vi "Cluster Terminal Get Elements Info.vi"(7 "skip first typedef?":bool, 8 "error in (no error)":errorcluster, 10 "ClusterConstant refnum":refnum<vi>, 11 "Terminal in":refnum<vi>) -> (0 "error out":errorcluster, 1 "is typedef?":bool, 2 "Cluster elements datatypes":string[](array[string]), 3 "Cluster elements names":string[](array[string]), 4 "typedef name":string)   [LabVIEW 2014]
doc: "Returns names and datatypes of elements inside cluster. If elemnet has no label, it's returned default name \"item0\" or \"item1\" or ... \"itemN\" which will be also used in generated code.\nIf wired Terminal then is used to get names and datatypes of ClusterConstant elements, otherwise is used ClusterConstant refnum."
uses:
  TranscriptorBasicObject.lvclass
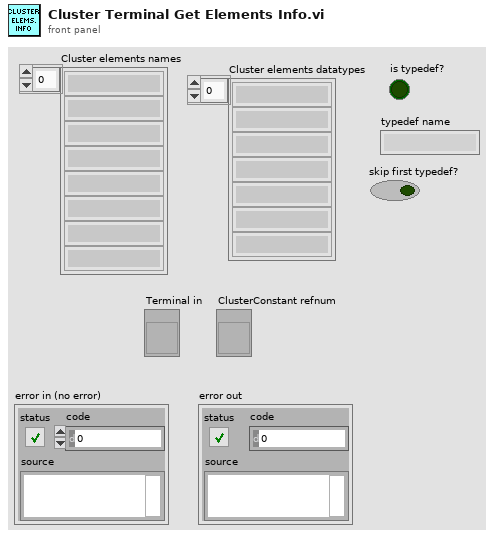
[diagram p1: front panel]
types:
  T1 = enum32{"not a typedef", "typedef", "strict typedef", "class private data"}[]
  T2 = enum32{"not a typedef", "typedef", "strict typedef", "class private data"}
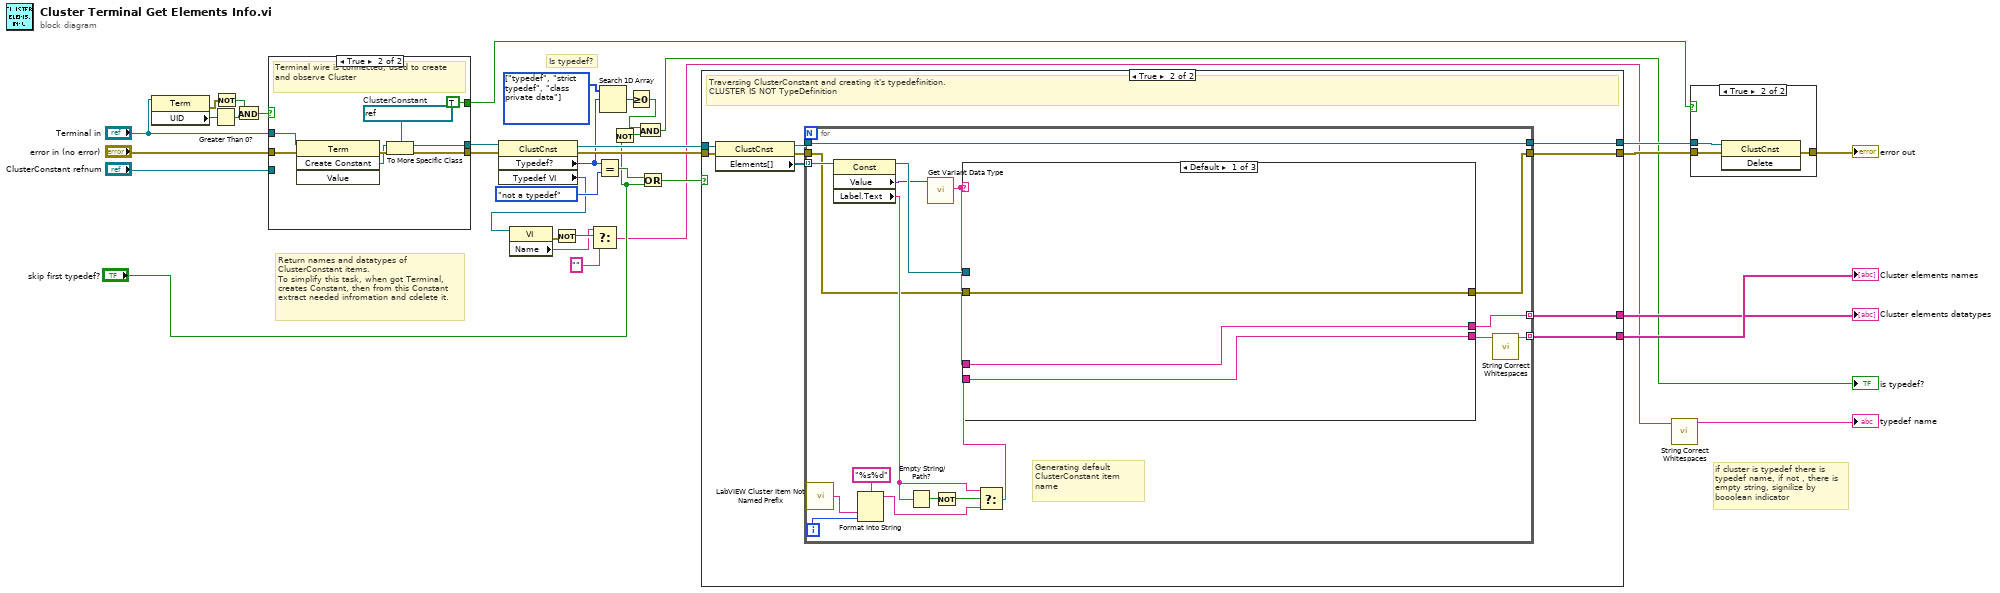
[diagram p0: block diagram]
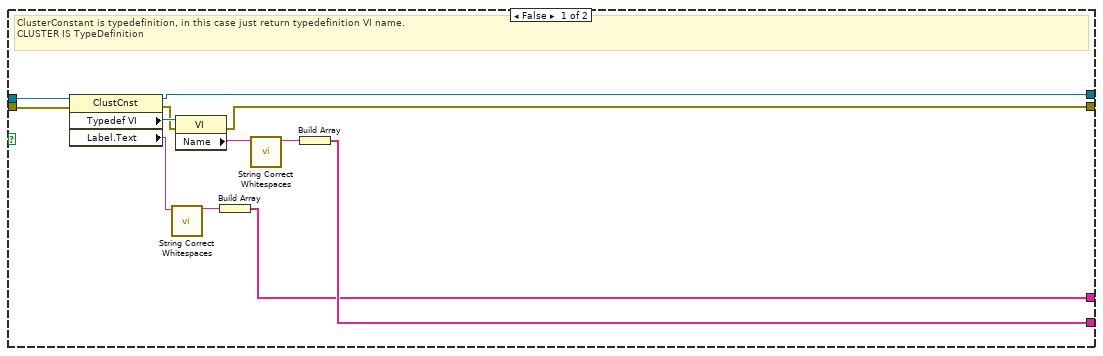
[diagram p2: hidden frame]
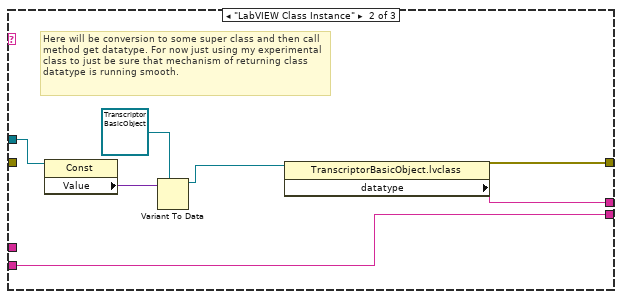
[diagram p3: hidden frame]
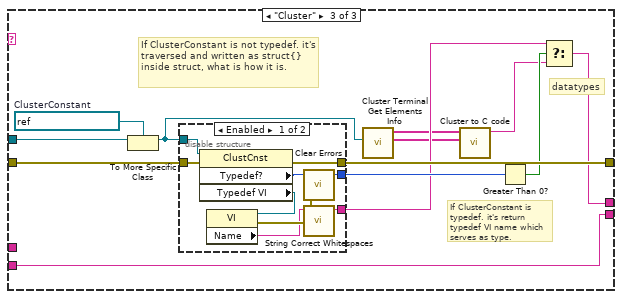
[diagram p4: hidden frame]
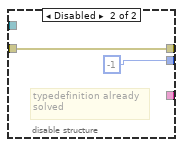
[diagram p5: hidden frame]
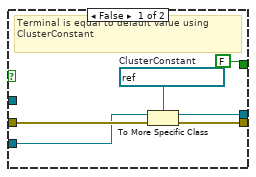
[diagram p7: hidden frame]
diagram:
  w16 = T1 [enum."typedef", enum."strict typedef", enum."class private data"] items=["not a typedef", "typedef", "strict typedef", "class private data"]
  # "if cluster is typedef there is typedef name, if not , there is empty string, signilize by booolean indicator"
  # "Is typedef?"
  # "Return names and datatypes of ClusterConstant items.\nTo simplify this task, when got Terminal, creates Constant, then from this Constant extract needed infromation and cdelete it."
  n1 = property class="Term"(reference="Terminal in") -> (error out=w20:errorcluster, "UID"=w22:i32)  [unwired: 1 in, 1 out]
  n2 = Greater Than 0?(x=w22) -> (x > 0?=w21:bool)
  n3 = Not(x=w20) -> (.not. x?=w19:bool)
  n4 = And(x=w19, y=w21) -> (x .and. y?=w18:bool)
  n5 = case shown="True" w18 {
    tunnel: [w39 w49] -> w28
    tunnel: "error in (no error)" -> [w38 w47]
    tunnel: [w40 w45] -> w29
    tunnel: "Terminal in" -> [_ w43]
    tunnel: [FALSE TRUE] -> w25
    tunnel: "ClusterConstant refnum" -> [w36 _]
    frame False {
      w41 = refnum<vi> refnum  # ClusterConstant
      # "Terminal is equal to default value using ClusterConstant"
      n6 = To More Specific Class(target class=w41, reference=w36, error in=w38) -> (specific class reference=w40:refnum<vi>, error out=w39:errorcluster)
    }
    frame True {
      w44 = refnum<vi> refnum  # ClusterConstant
      # "Terminal wire is connected, used to create and observe Cluster"
      n7 = invoke on="Invoke Node" class="Term" method="Create Constant"(reference=w43, error in=w47) -> (error out=w48:errorcluster, "Create Constant"=w46:refnum<vi>)  [unwired: 2 in, 2 out]
      n8 = To More Specific Class(target class=w44, reference=w46, error in=w48) -> (specific class reference=w45:refnum<vi>, error out=w49:errorcluster)
    }
  }
  n9 = property on="Property Node" class="ClustCnst"(reference=w29, error in=w28) -> (reference out=w27:refnum<vi>, error out=w26:errorcluster, "Typedef?"=w15:T2, "Typedef VI"=w7:refnum<vi>)
  n10 = property on="Property Node" class="VI"(reference=w7) -> (error out=w6:errorcluster, "Name"=w4:string)  [unwired: 1 in, 1 out]
  n11 = Not(x=w6) -> (.not. x?=w5:bool)
  n12 = Select(t=w4, s=w5, f="") -> (s? t:f=w2:string)
  n13 = Equal?(x=w15, y=T2."not a typedef" ("Is Typedef?")) -> (x = y?=w13:bool)
  n14 = Search 1D Array(1D array=w16, element=w15) -> (index of element=w14:i32)  [unwired: 1 in]
  n15 = Not(x="skip first typedef?") -> (.not. x?=w8:bool)
  n16 = Greater Or Equal To 0?(x=w14) -> (x >= 0?=w11:bool)
  n17 = And(x=w11, y=w8) -> (x .and. y?=→"is typedef?":bool)
  n18 = Or(x=w13, y="skip first typedef?") -> (x .or. y?=w12:bool)
  n19 = case shown="True" w12 {
    tunnel: [w55 w70] -> w34
    tunnel: w26 -> [w60 w68]
    tunnel: w27 -> [w61 w66]
    tunnel: [w57 w64] -> w32
    tunnel: [w53 w63] -> w31
    tunnel: [w52 w62] -> w30
    frame False {
      # "ClusterConstant is typedefinition, in this case just return typedefinition VI name.\nCLUSTER IS TypeDefinition"
      n20 = property on="Property Node" class="ClustCnst"(reference=w61, error in=w60) -> (reference out=w57:refnum<vi>, error out=w56:errorcluster, "Typedef VI"=w59:refnum<vi>, "Label.Text"=w51:string)
      n21 = call "String Correct Whitespaces.vi"("String in"=w51) -> ("String out"=w50:string)  [unwired: 10 in]
      n22 = property on="Property Node" class="VI"(reference=w59, error in=w56) -> (error out=w55:errorcluster, "Name"=w58:string)  [unwired: 1 out]
      n23 = Build Array(w50) -> (w52:string[])
      n24 = call "String Correct Whitespaces.vi"("String in"=w58) -> ("String out"=w54:string)  [unwired: 10 in]
      n25 = Build Array(w54) -> (w53:string[])
    }
    frame True {
      # "Traversing ClusterConstant and creating it's typedefinition.\nCLUSTER IS NOT TypeDefinition"
      n26 = property on="Property Node" class="ClustCnst"(reference=w66, error in=w68) -> (reference out=w65:refnum<vi>, error out=w69:errorcluster, "Elements[]"=w67:refnum<vi>[])
      n27 = for {
        tunnel: w67 -> [w88] mode=indexing
        tunnel: w69 -> [w79]
        tunnel: [w78] -> w70
        tunnel: w65 -> [w80]
        tunnel: [w80] -> w64
        tunnel: [w75] -> w62 mode=indexing
        tunnel: [w72] -> w63 mode=indexing
        i -> [w83]
        # "Generating default ClusterConstant item name"
        n28 = call "LabVIEW Cluster Item Not Named Prefix.vi"() -> ("not named cluster item prefix"=w82:string)
        n29 = property class="Const"(reference=w88) -> (reference out=w76:refnum<vi>, "Value"=w73:variant, "Label.Text"=w81:string)  [unwired: 1 in, 1 out]
        n30 = Format Into String(format string="%s%d", w82, w83) -> (resulting string=w84:string)  [unwired: 2 in, 1 out]
        n31 = Empty String/Path?(string/path=w81) -> (empty?=w87:bool)
        n32 = call "Get Variant Data Type.vi"("Variant in"=w73) -> ("first data type"=w74:string)  [unwired: 9 in, 1 out]
        n33 = Not(x=w87) -> (.not. x?=w86:bool)
        n34 = Select(t=w81, s=w86, f=w84) -> (s? t:f=w77:string)
        n35 = case shown="Default" w74 {
          tunnel: w76 -> [_ w95 w99]
          tunnel: w79 -> [w91 _ w110]
          tunnel: [w91 w96 w108] -> w78
          tunnel: w77 -> [w89 w97 w105]
          tunnel: w74 -> [w90 _ _]
          tunnel: [w90 w98 w107] -> w75
          tunnel: [w89 w97 w105] -> w71
          frame Default {
          }
          frame "LabVIEW Class Instance" {
            # "Here will be conversion to some super class and then call method get datatype. For now just using my experimental class to just be sure that mechanism of returning class datatype is running smooth."
            n36 = property class="Const"(reference=w95) -> ("Value"=w94:variant)  [unwired: 1 in, 2 out]
            n37 = Variant To Data(type=refnum<class "TranscriptorBasicObject.lvclass"> refnum ("TranscriptorBasicObject.lvclass"), Variant=w94) -> (data=w93:refnum<class "TranscriptorBasicObject.lvclass">)  [unwired: 1 in, 1 out]
            n38 = property class="TranscriptorBasicObject.lvclass"(reference=w93) -> (error out=w96:errorcluster, "datatype"=w98:string)  [unwired: 1 in, 1 out]
          }
          frame "Cluster" {
            w111 = refnum<vi> refnum  # ClusterConstant
            # "If ClusterConstant is typedef. it's return typedef VI name which serves as type."
            # "If ClusterConstant is not typedef. it's traversed and written as struct{} inside struct, what is how it is."
            # "datatypes"
            n39 = To More Specific Class(target class=w111, reference=w99) -> (specific class reference=w100:refnum<vi>)  [unwired: 1 in, 1 out]
            n40 = disable-structure shown="Enabled" {
              disable-tunnel: w110 -> [w119 w121]
              disable-tunnel: [w118 -1] -> w109
              disable-tunnel: [w114 w121] -> w108
              disable-tunnel: [w113 _] -> w104
              disable-tunnel: w100 -> [w112 _]
              frame Enabled {
                n41 = property class="ClustCnst"(reference=w112, error in=w119) -> (error out=w114:errorcluster, "Typedef?"=w118:T2, "Typedef VI"=w115:refnum<vi>)  [unwired: 1 out]
                n42 = property class="VI"(reference=w115) -> (error out=w117:errorcluster, "Name"=w116:string)  [unwired: 1 in, 1 out]
                n43 = call <vilib>:"Clear Errors.vi"("error in (no error)"=w117) -> ()  [unwired: 5 in, 2 out]
                n44 = call "String Correct Whitespaces.vi"("String in"=w116) -> ("String out"=w113:string)  [unwired: 10 in]
              }
              frame Disabled {
                # "typedefinition already\nsolved"
              }
            }
            n45 = call "Cluster Terminal Get Elements Info.vi"("ClusterConstant refnum"=w100) -> ("Cluster elements datatypes"=w102:string[], "Cluster elements names"=w103:string[])  [unwired: 6 in, 3 out]
            n46 = call "Cluster to C code.vi"("Cluster elements datatypes"=w102, "Cluster elements names"=w103) -> ("C code"=w101:string)  [unwired: 9 in]
            n47 = Greater Than 0?(x=w109) -> (x > 0?=w106:bool)
            n48 = Select(t=w104, s=w106, f=w101) -> (s? t:f=w107:string)
          }
        }
        n49 = call "String Correct Whitespaces.vi"("String in"=w71) -> ("String out"=w72:string)  [unwired: 10 in]
      }
    }
  }
  "Cluster elements datatypes" <- w30
  "Cluster elements names" <- w31
  n50 = call "String Correct Whitespaces.vi"("String in"=w2) -> ("String out"=→"typedef name":string)  [unwired: 10 in]
  n51 = case shown="True" w25 {
    tunnel: [w122 w125] -> w35
    tunnel: w34 -> [w122 w124]
    tunnel: w32 -> [_ w123]
    frame False {
    }
    frame True {
      n52 = invoke on="Invoke Node" class="ClustCnst" method="Delete"(reference=w123, error in=w124) -> (error out=w125:errorcluster)  [unwired: 1 in, 2 out]
    }
  }
  "error out" <- w35
